vi "read_buff.vi"(9 "buffer":string) -> ()   [LabVIEW 2016]
uses:
  <vilib>/regexp/Match Regular Expression.xnode
panel:
  out "error out queue2":errorcluster
  out "error out queue1":errorcluster
  out "result string":string
  out "array":string[](array[string])
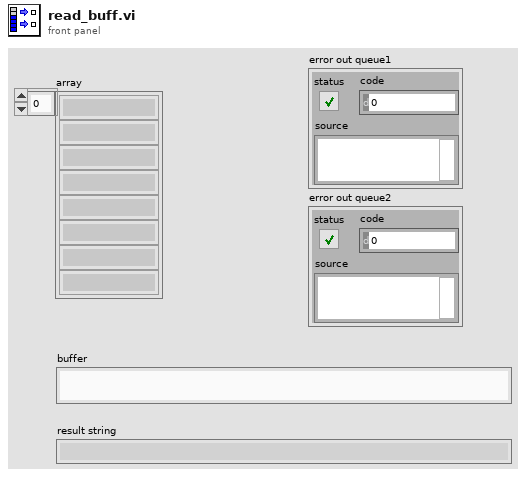
[diagram p1: front panel]
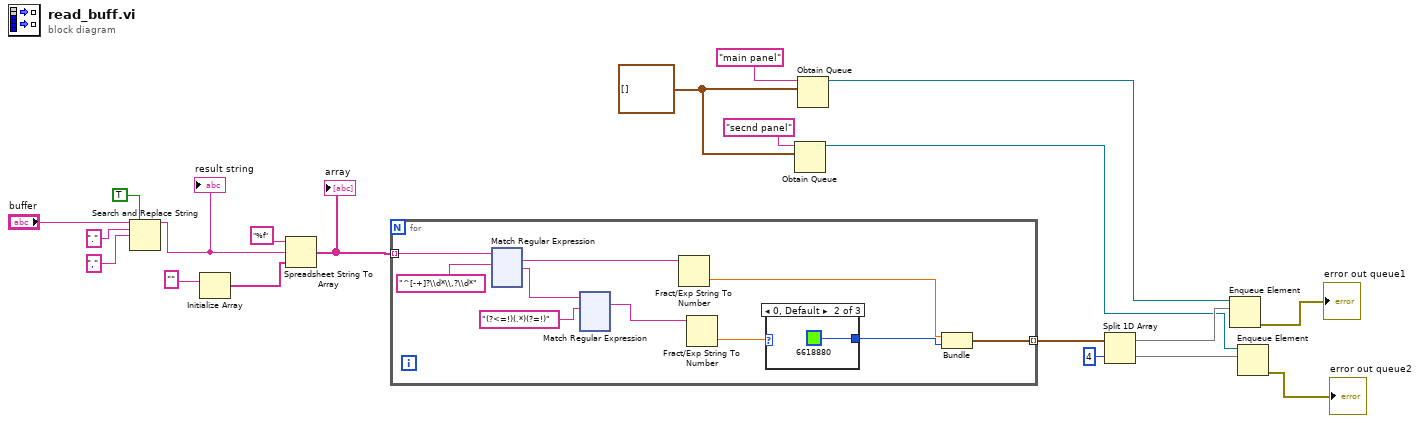
[diagram p0: block diagram]
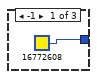
[diagram p2: hidden frame]
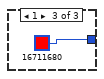
[diagram p3: hidden frame]
diagram:
  w5 = cluster{dbl, "Round Color Box":u32}[] []
  n1 = Search and Replace String(replace all?=TRUE ("replace all? (F)"), input string="buffer", search string="." ("replace string (\"\")"), replace string="," ("replace string (\"\")")) -> (result string=w17:string)  [unwired: 4 in, 3 out]
  "result string" <- w17
  n2 = Initialize Array("") -> (w14:string[])  [unwired: 1 in]
  n3 = Spreadsheet String To Array(format string="%f", spreadsheet string=w17, array type (2D Dbl)=w14) -> (array=w12:string[])  [unwired: 1 in]
  "array" <- w12
  n4 = for {
    tunnel: w12 -> [w29] mode=indexing
    tunnel: [w22] -> w9 mode=indexing
    n5 = xnode "Match Regular Expression"("input string"=w29, "regular expression"="^[-+]?\\d*\\,?\\d*") -> ("whole match"=w26:string, "after match"=w27:string)  [unwired: 4 in, 3 out]
    n6 = xnode "Match Regular Expression"("input string"=w27, "regular expression"="(?<=!)(.*)(?=!)") -> ("whole match"=w25:string)  [unwired: 4 in, 4 out]
    n7 = Fract/Exp String To Number(string=w26) -> (number=w23:dbl)  [unwired: 3 in, 1 out]
    n8 = Fract/Exp String To Number(string=w25) -> (number=w21:dbl)  [unwired: 3 in, 1 out]
    n9 = case shown="0, Default" w21 {
      tunnel: [u32 16772608 ("Round Color Box") u32 6618880 ("Round Color Box") u32 16711680 ("Round Color Box")] -> w24
      frame -1 {
      }
      frame 0, Default {
      }
      frame 1 {
      }
    }
    n10 = Bundle(w23, "Round Color Box"=w24) -> (w22:cluster{dbl, "Round Color Box":u32})  [unwired: 1 in]
  }
  n11 = Obtain Queue(name (unnamed)="secnd panel", element data type=w5) -> (queue out=w3:refnum<queue>)  [unwired: 3 in, 2 out]
  n12 = Obtain Queue(name (unnamed)="main panel", element data type=w5) -> (queue out=w4:refnum<queue>)  [unwired: 3 in, 2 out]
  n13 = Split 1D Array(array=w9, index=4) -> (first subarray=w6:cluster{dbl, "Round Color Box":u32}[], second subarray=w7:cluster{dbl, "Round Color Box":u32}[])
  n14 = Enqueue Element(queue=w4, element=w6) -> (error out=→"error out queue1":errorcluster)  [unwired: 2 in, 2 out]
  n15 = Enqueue Element(queue=w3, element=w7) -> (error out=→"error out queue2":errorcluster)  [unwired: 2 in, 2 out]
